vi "update digital outputs.vi"(9 "Message handler data":T1, 11 "Data":variant) -> (0 "error":errorcluster)   [LabVIEW 2018]
uses:
  Type Defs/Message loop data.ctl
  Type Defs/FPGA reference.ctl
  Type Defs/RT Status.ctl
  <vilib>/Utility/error.llb/Error Cluster From Error Code.vi
  <vilib>/rvi/errors/niLvFpgaAdjustHostInterfaceError.vi
  <vilib>/rvi/interface/nirviReadWriteControl/nirviReadWriteControl.xnode
  FPGA Bitfiles/CompressorRigV2_CompressorFPGA_FPGAMainV3_7sPRekuravM.lvbitx
  NiFpgaLv.dll
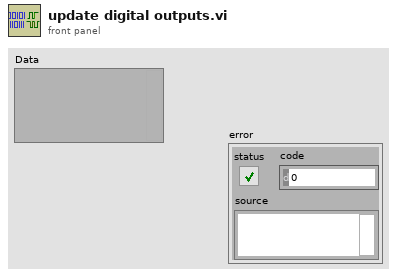
[diagram p1: front panel]
types:
  T1 = typedef "Message loop data.ctl" = cluster{"Parameters":cluster{"FPGA Ref":T2, "configID":u32, "activeChannels":cluster{"index":u16, "name":string}[]}, "Variables":cluster{"RT Status":T3, "watchdog":timestamp, "limitsEnabled":bool, "Interlocks":cluster{"gearboxOil":bool, "bearingOil":bool, "gearboxAir":bool}}}
  T2 = typedef "FPGA reference.ctl" = refnum<k20>
  T3 = typedef "RT Status.ctl" = cluster{"Comms loop":bool, "scheduler loop":bool, "data process loop":bool, "FIFO loop":bool, "Command Stream":bool, "Error Stream":bool, "FPGA FIFO":bool, "Data Stream":bool}
  T4 = cluster{"new output":bool, "module":enum16{"7", "8"}, "Index":i32}
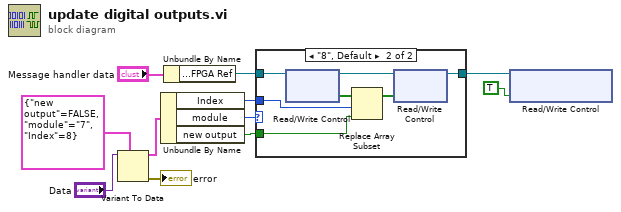
[diagram p0: block diagram]
diagram:
  n1 = Variant To Data(type=T4 {"new output"=FALSE, "module"=enum."7", "Index"=8}, Variant="Data") -> (data=w7:T4, error out=→"error":errorcluster)  [unwired: 1 in]
  n2 = Unbundle By Name(w7) -> ("Index"=w2:i32, "module"=w3:enum16{"7", "8"}, "new output"=w4:bool)
  n3 = Unbundle By Name("Message handler data") -> ("Parameters.FPGA Ref"=w10:T2)
  n4 = case shown="\"8\", Default" w3 {
    tunnel: w10 -> [w12 w19]
    tunnel: [w12 w17] -> w6
    tunnel: w4 -> [_ w13]
    tunnel: w2 -> [_ w14]
    frame "7" {
    }
    frame "8", Default {
      n5 = xnode "Read/Write Control"("FPGA VI Reference In"=w19) -> ("FPGA VI Reference Out"=w18:T2, "Mod 8"=w16:bool[])  [unwired: 1 in, 1 out]
      n6 = Replace Array Subset(array=w16, new element=w13, index=w14) -> (w15:bool[])
      n7 = xnode "Read/Write Control"("FPGA VI Reference In"=w18, "Mod 8"=w15) -> ("FPGA VI Reference Out"=w17:T2)  [unwired: 1 in, 1 out]
    }
  }
  n8 = xnode "Read/Write Control"("FPGA VI Reference In"=w6, "Update Outputs"=TRUE ("Enable Data FIFO")) -> ()  [unwired: 1 in, 2 out]
